vi "Create Empty.vi"(8 "error in (no error)":errorcluster) -> (0 "error out":errorcluster, 3 "Empty Buffer":refnum<class "Buffer.lvclass">)   [LabVIEW 2020, in "Buffer.lvclass"]
uses:
  Buffer.lvclass
  Buffer.lvclass/Buffer.ctl
  bin/gindustrialcam_32-1.dll
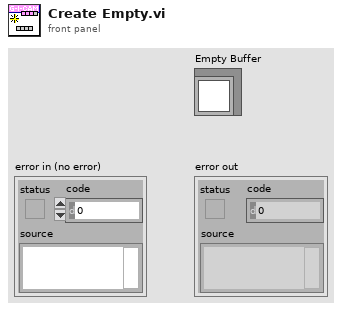
[diagram p1: front panel]
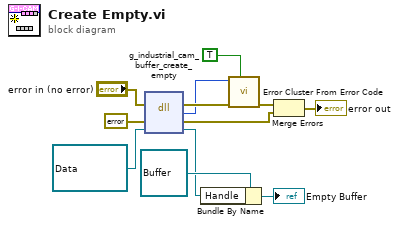
[diagram p0: block diagram]
diagram:
  n1 = dll-call lib="C:/serenial/lib/g-industrial-camera/LabVIEW/g_industrial_cam/bin/gindustrialcam_*-1.*" fn="g_industrial_cam_buffer_create_empty"(error in="error in (no error)", "err"=errorcluster {"status"=FALSE, "code"=0, "source"=""} ("error constant"), "edvr"=refnum<data-value> refnum ("Handle")) -> (error out=w10:errorcluster, "Mg_Error"=w9:i32, "err"=w7:errorcluster, "edvr"=w1:refnum<data-value>)  [unwired: 2 in, 1 out]
  n2 = Bundle By Name(cluster=refnum<class "Buffer.lvclass"> refnum ("Buffer in"), "Handle"=w1) -> (→"Empty Buffer":refnum<class "Buffer.lvclass">)
  n3 = call <vilib>:"Error Cluster From Error Code.vi"("show call chain? (False)"=TRUE, "error in (no error)"=w10, "error code (0)"=w9) -> ("error out"=w8:errorcluster)  [unwired: 6 in]
  n4 = Merge Errors(w8, w7) -> (→"error out":errorcluster)
